vi "ClearFIFO.vi"(8 "error in (no error)":errorcluster) -> (0 "error out":errorcluster)   [LabVIEW 2012]
doc: "unsigned long AIOUSB_ClearFIFO(\nunsigned long DeviceIndex - number from 0-31 of the device you wish to clear the streaming\nFIFO on.\nunsigned long Method - 0 to simply clear the FIFO right away, others per the table below\n)\nThis function is only supported by boards with large input FIFOs - that is, the USB-AIxx-xxx\nseries, USB-DI-16A, and USB-DIO16-16A.\nClear FIFO Method Codes\nCode\n(decimal) Effect\n0 Clear FIFO as soon as command received\n1 Clear FIFO on next REN disable edge (on digital boards, analog boards treat as 0)\n5 Clear FIFO and abort stream (analog boards only)\n86 As 1, but also wait until that edge (on digital boards, analog boards treat as 0)\nAll DWORD return values other than GetDevices() are Windows Error Codes and return\n\"ERROR_SUCCESS\" (equal to 0) if no error occurred. If the USB device has been removed\nduring use, the error returned is \"ERROR_DEVICE_REMOVED\" (equal to 1617 decimal) and\nwill persist until a call toQueryDeviceInfo() with non-null pNameSize has been made for that\ndevice. If this state is cleared and the board was not reconnected, the error returned is\n27\n\"ERROR_FILE_NOT_FOUND\" (equal to 2). Versions of AIOUSB.dll prior to 2.1 return\n\"ERROR_DEV_NOT_EXIST\" (equal to 55 decimal) under both conditions.\nThe constants diFirst (equal to FFFFFFFE hex) and diOnly (equal to FFFFFFFD hex) can be\npassed for DeviceIndex in place of an actual device index. diFirst causes the function to operate\non the first device, whatever its device index. diOnly causes the function to operate on the only\ndevice if there is only one, or to return \"ERROR_DUP_NAME\" (equal to 52 decimal) if there's\nmore than one device."
uses:
  Controls/AIOUSB_ClearFIFO.ctl
  Windows/System32/AIOUSB.dll
panel:
  in  "Method":T1 items=["Clear now"=0, "Clear on Next REN edge"=1, "Clear and About Stream"=5, "Clear on this REN edge"=86]
  in  "DeviceIndex":u32
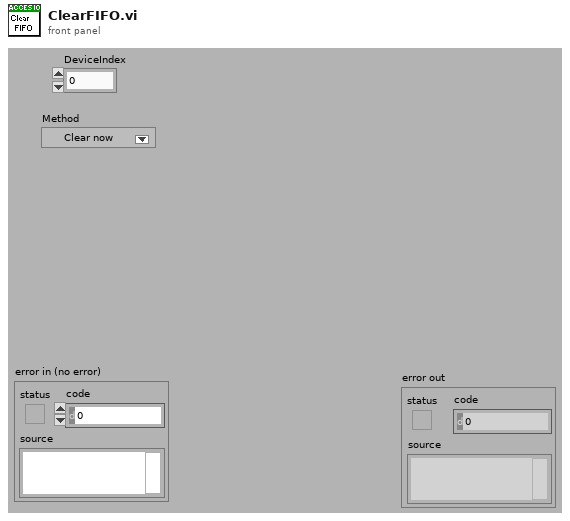
[diagram p1: front panel]
types:
  T1 = typedef "AIOUSB_ClearFIFO.ctl" = u16
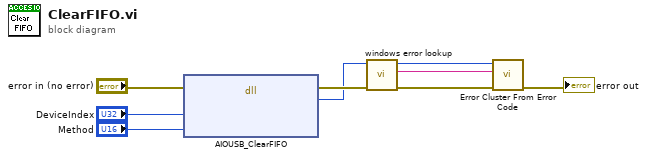
[diagram p0: block diagram]
diagram:
  n1 = dll-call lib="C:/Windows/System32/AIOUSB.dll" fn="AIOUSB_ClearFIFO"(error in="error in (no error)", "DeviceIndex"="DeviceIndex", "Method"="Method") -> (error out=w3:errorcluster, "return type"=w1:u32)  [unwired: 4 in, 1 out]
  n2 = call "windows error lookup.vi"("error in (no error)"=w3, "Error Code"=w1) -> ("error out"=w2:errorcluster, "error message (\"\")"=w4:string)  [unwired: 8 in]
  n3 = call <vilib>:"Error Cluster From Error Code.vi"("error in (no error)"=w2, "error message (\"\")"=w4, "error code (0)"=w1) -> ("error out"=→"error out":errorcluster)  [unwired: 6 in]
